vi "read_4ch.vi"(10 "channel offsets":T1, 11 "converter box version":i16=1 min=1 max=2) -> (2 "read output":T1)   [LabVIEW 2010]
uses:
  common_typedefs/channels_cluster.ctl
  common_typedefs/channel_decoding_enum.ctl
  <vilib>/eio/EIONode/EIONode.xnode
  <vilib>/rvi/eio/nirviEIOImplementation/nirviEIOImplementation.xnode
  <vilib>/rvi/eio/common/nirviEmuClasses.ctl
  <vilib>/rvi/eio/common/nirviEmuTemplateMethod_noerrors.vi
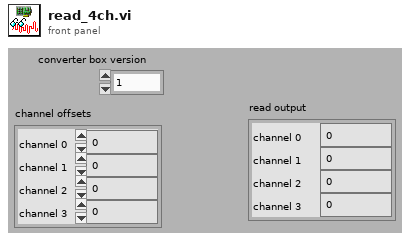
[diagram p1: front panel]
types:
  T1 = typedef "channels_cluster.ctl" = cluster{"channel 0":u32, "channel 1":u32, "channel 2":u32, "channel 3":u32}
  T2 = typedef "channel_decoding_enum.ctl" = enum16{"A", "B"}
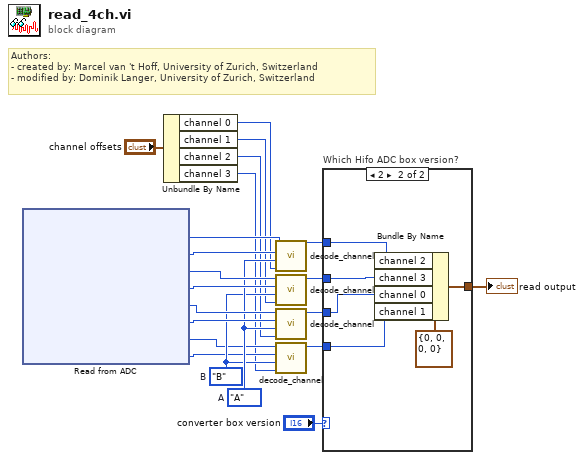
[diagram p0: block diagram]
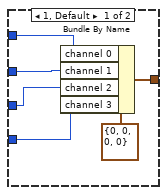
[diagram p2: hidden frame]
diagram:
  w11 = channel_decoding_enum."B"  # B
  w12 = channel_decoding_enum."A"  # A
  # "Authors: \n- created by: Marcel van 't Hoff, University of Zurich, Switzerland\n- modified by: Dominik Langer, University of Zurich, Switzerland"
  n1 = xnode "Read from ADC"() -> ("Connector1/DIOPORT3"=w19:u8, "Connector1/DIOPORT2"=w18:u8, "Connector1/DIOPORT1"=w16:u8, "Connector1/DIOPORT0"=w15:u8, "Connector0/DIOPORT3"=w14:u8, "Connector0/DIOPORT2"=w13:u8, "Connector0/DIOPORT1"=w10:u8, "Connector0/DIOPORT0"=w9:u8)  [unwired: 8 in, 8 out]
  n2 = Unbundle By Name("channel offsets") -> ("channel 0"=w5:u32, "channel 1"=w4:u32, "channel 2"=w3:u32, "channel 3"=w2:u32)
  n3 = call "decode_channel.vi"("offset"=w5, "channel decoding"=w12, "port B"=w18, "port A"=w19) -> ("channel value"=w17:u32)  [unwired: 7 in]
  n4 = call "decode_channel.vi"("offset"=w4, "channel decoding"=w11, "port B"=w15, "port A"=w16) -> ("channel value"=w8:u32)  [unwired: 7 in]
  n5 = call "decode_channel.vi"("offset"=w3, "channel decoding"=w12, "port B"=w13, "port A"=w14) -> ("channel value"=w7:u32)  [unwired: 7 in]
  n6 = call "decode_channel.vi"("offset"=w2, "channel decoding"=w11, "port B"=w9, "port A"=w10) -> ("channel value"=w6:u32)  [unwired: 7 in]
  n7 = case "Which Hifo ADC box version?" shown="2" "converter box version" {
    tunnel: w17 -> [w27 w33]
    tunnel: w8 -> [w26 w32]
    tunnel: w7 -> [w25 w31]
    tunnel: w6 -> [w24 w30]
    tunnel: [w23 w28] -> w1
    frame 1, Default {
      n8 = Bundle By Name(cluster=T1 {"channel 0"=0, "channel 1"=0, "channel 2"=0, "channel 3"=0} ("channel offsets 3"), "channel 0"=w27, "channel 1"=w26, "channel 2"=w25, "channel 3"=w24) -> (w23:T1)
    }
    frame 2 {
      n9 = Bundle By Name(cluster=T1 {"channel 0"=0, "channel 1"=0, "channel 2"=0, "channel 3"=0} ("channel offsets 3"), "channel 2"=w33, "channel 3"=w32, "channel 0"=w31, "channel 1"=w30) -> (w28:T1)
    }
  }
  "read output" <- w1
